vi "Camera-Cluster2Device.vi"(4 "Camera Device IN":T1) -> (0 "Error OUT":errorcluster, 1 "hCamera OUT":u32, 2 "uSerialNumber OUT":u32)   [LabVIEW 2010]
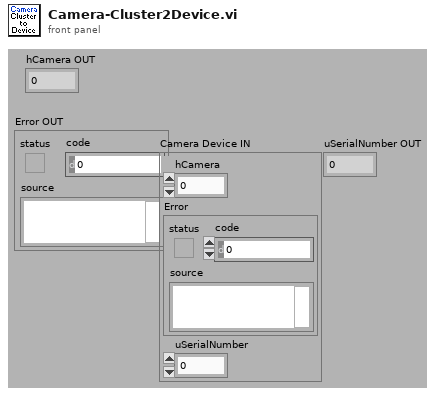
[diagram p1: front panel]
types:
  T1 = cluster{"hCamera":u32, "Error":errorcluster, "uSerialNumber":u32}
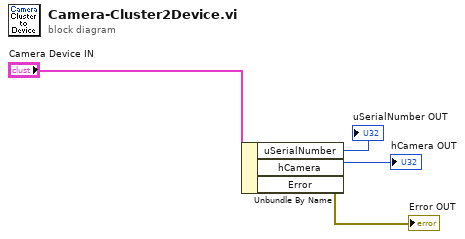
[diagram p0: block diagram]
diagram:
  n1 = Unbundle By Name("Camera Device IN") -> ("uSerialNumber"=→"uSerialNumber OUT":u32, "hCamera"=→"hCamera OUT":u32, "Error"=→"Error OUT":errorcluster)
